vi "Sine wave.vi"() -> ()   [LabVIEW 2020]
uses:
  <vilib>/Analysis/NI_AALBase.lvlib
panel:
  in  "Scale":dbl=1.0 format="%#_13g"
  out "웨이브폼 그래프":i8[][](graph)
  in  "PWM":i32=48000
  in  "Freq":i32=160
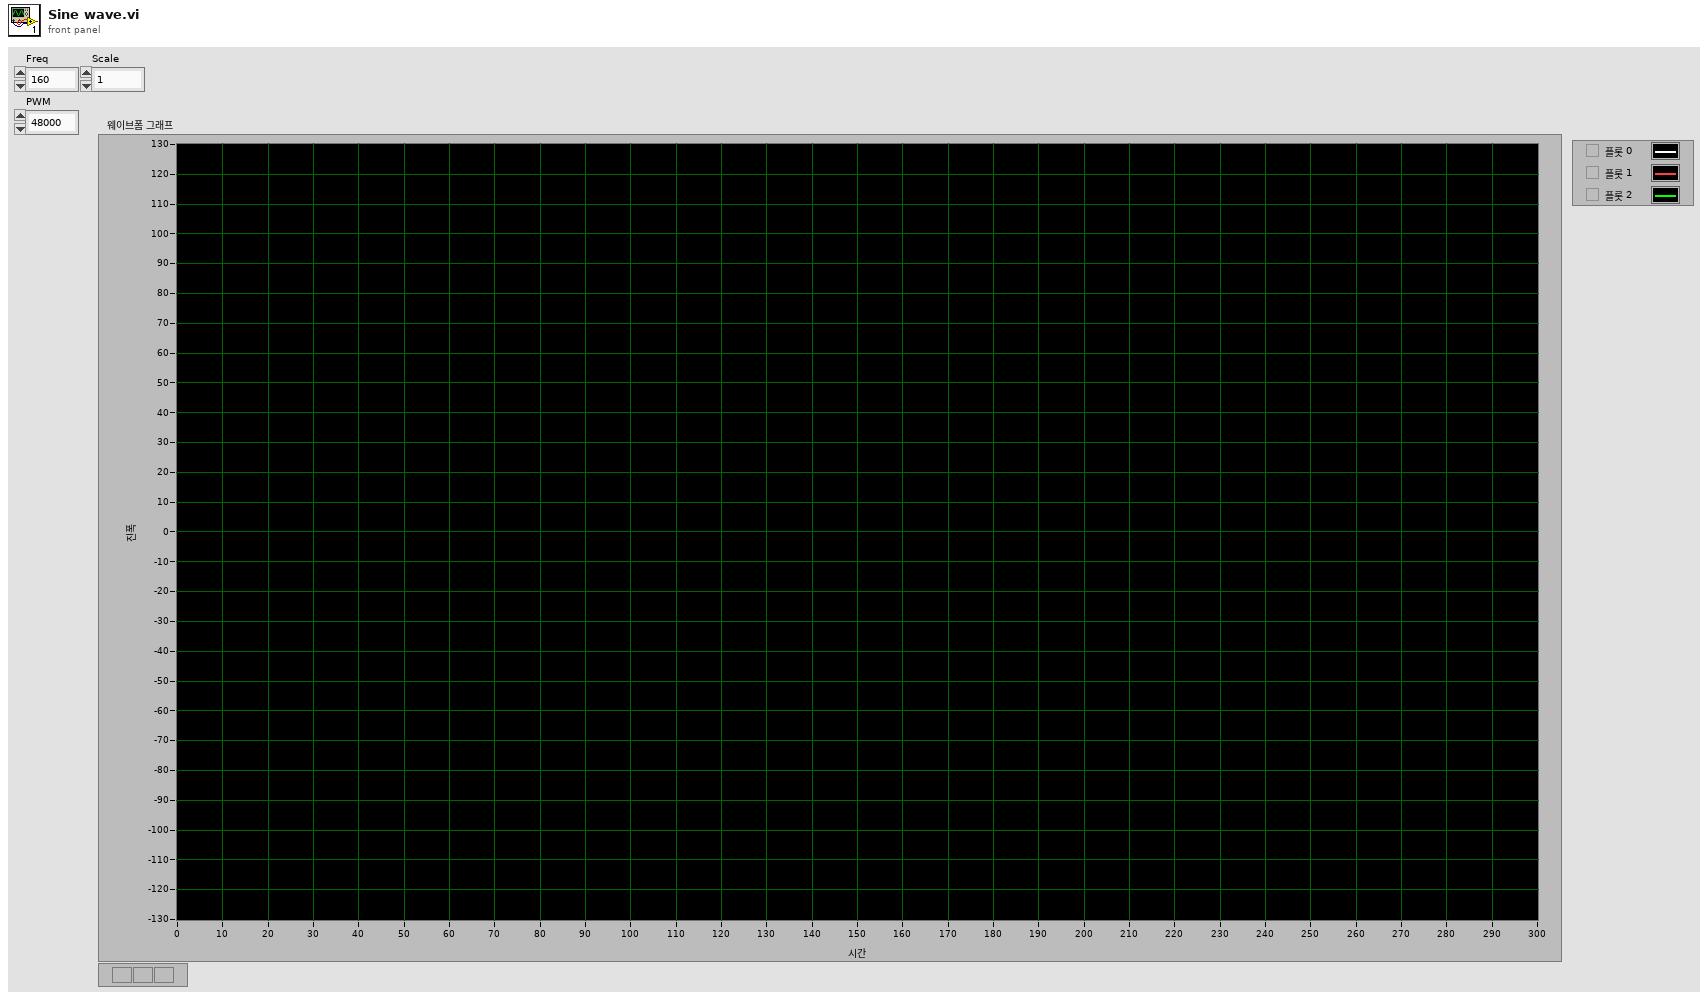
[diagram p1: front panel]
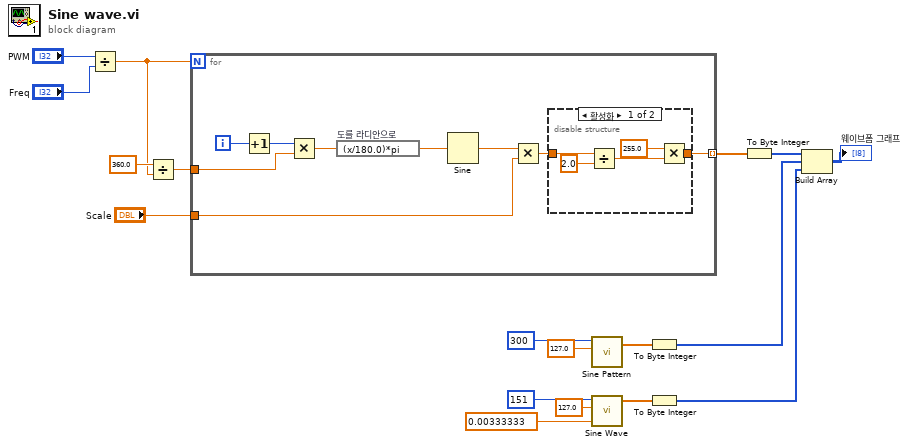
[diagram p0: block diagram]
diagram:
  n1 = Divide(x="PWM", y="Freq") -> (x/y=w16:dbl)
  n2 = Divide(x=360.0, y=w16) -> (x/y=w15:dbl)
  n3 = for {
    N: w16 -> [_]
    tunnel: w15 -> [w24]
    tunnel: [w21] -> w14 mode=indexing
    tunnel: "Scale" -> [w22]
    i -> [w20]
    n4 = Increment(x=w20) -> (x+1=w19:i32)
    n5 = Multiply(x=w19, y=w24) -> (x*y=w25:dbl)
    n6 = expression code="(x/180.0)*pi" "도를 라디안으로"(w25) -> (w27:dbl)
    n7 = Sine(x=w27) -> (sin(x)=w26:dbl)
    n8 = Multiply(x=w26, y=w22) -> (x*y=w23:dbl)
    n9 = disable-structure shown="활성화" {
      disable-tunnel: w23 -> [w32 w33]
      disable-tunnel: [w29 w33] -> w21
      frame Enabled {
        n10 = Divide(x=w32, y=2.0) -> (x/y=w31:dbl)
        n11 = Multiply(x=255.0, y=w31) -> (x*y=w29:dbl)
      }
      frame Disabled {
      }
    }
  }
  n12 = call <vilib>:"Sine Pattern.vi"("amplitude"=127.0, "samples"=300) -> ("Sinusoidal Pattern"=w9:dbl[])  [unwired: 2 in, 1 out]
  n13 = call <vilib>:"Sine Wave.vi"("samples"=151, "amplitude"=127.0, "frequency"=0.00333333) -> ("sine wave"=w3:dbl[])  [unwired: 2 in, 2 out]
  n14 = To Byte Integer(number=w9) -> (8bit integer=w7:i8[])
  n15 = To Byte Integer(number=w3) -> (8bit integer=w2:i8[])
  n16 = To Byte Integer(number=w14) -> (8bit integer=w12:i8[])
  n17 = Build Array(w12, w7, w2) -> (→"웨이브폼 그래프":i8[][])
